vi "Config CCD.vi"(8 "error in (no error)":errorcluster, 11 "Configuration in":refnum<class "Configuration.lvclass">) -> (0 "error out":errorcluster, 3 "Configuration out":refnum<class "Configuration.lvclass">)   [LabVIEW 2016, in "CCD.lvlib" / "CCD Configuration.lvclass"]
uses:
  <userlib>/Common Components/Hardware/CCD/CCD Configuration.lvclass
  <userlib>/Configuration Dialog Actor/Configuration.lvclass
  <userlib>/Common Components/Hardware/CCD/CCD/camer data.ctl
  C:/Program Files (x86)/National Instruments/LabVIEW 2016/user.lib/Configuration Dialog Actor/Configuration.lvclass
  <userlib>/Common Components/Hardware/CCD/CCD Configuration.lvclass/CCD Configuration.ctl
  <userlib>/Common Components/Hardware/Abstract Hardware/Hardware.lvclass/Hardware.ctl
  <userlib>/Common Components/Hardware/CCD/CCD/CCD.lvclass/CCD.ctl
  <userlib>/Common Components/Hardware/DevInfo/DevInfo.lvclass/DevInfo.ctl
  <userlib>/Common Components/Hardware/Abstract Hardware/Read DevInfo.vi
  <userlib>/Common Components/Hardware/DevInfo/Read COMM Address.vi
  <userlib>/Common Components/Hardware/DevInfo/Read Sub-COMM Address.vi
  <userlib>/Common Components/Hardware/DevInfo/Read HW Type.vi
  <userlib>/Common Components/Hardware/DevInfo/Read Device Name.vi
  <userlib>/Common Components/Hardware/DevInfo/Read Status.vi
  <userlib>/Common Components/Hardware/CCD/CCD/CCD.lvclass
  C:/Program Files (x86)/National Instruments/LabVIEW 2016/user.lib/Common Components/Hardware/Abstract Hardware/Hardware.lvclass
  <userlib>/Common Components/Hardware/DevInfo/DevInfo.lvclass
panel:
  in  "Cluster":T1={"VideoMode"=0, "gain"=6818, "gamma"=0.43, "Contrast"=37.81818181818181, "Exposure"=32, "Saturation"=6818} {"Saturation" max=7764 scale=0.0..7764.0; "Exposure" scale=1.0..2048.0; "Contrast" min=0.0 max=78.0 scale=0.0..78.0 scale format="%.2f"; "gamma" min=0.43 max=5 scale=0.43..5.0; "gain" min=1000 max=7000 scale=1000.0..7000.0; "VideoMode" items=["640x480 RGB24 30FPS", "1024x768 RGB24 18FPS", "1920x1080 RGB24  10FPS", "2048x1536 RGB24 3FPS"]}
  out "Status":bool
  out "HW Type":string
  out "Sub-COMM Address":string
  out "COMM Address":string
  out "Device Name":string
  in  "Revert":bool
  in  "Apply":bool
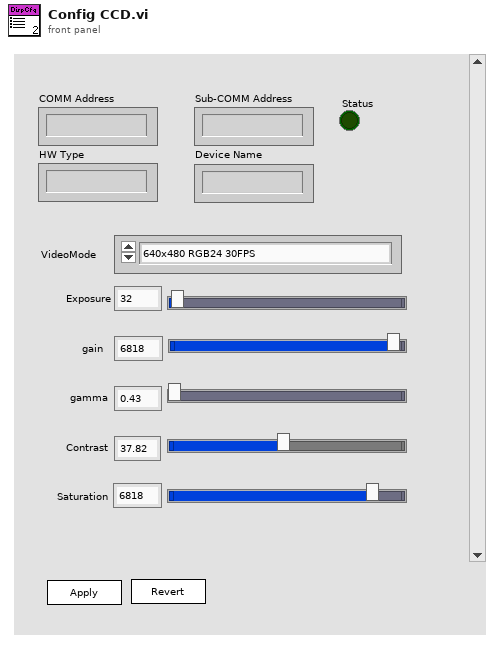
[diagram p1: front panel]
types:
  T1 = typedef "CCD.lvlib/CCD.lvclass/camer data.ctl" = cluster{"VideoMode":u16, "gain":u32, "gamma":sgl, "Contrast":dbl, "Exposure":u32, "Saturation":u32}
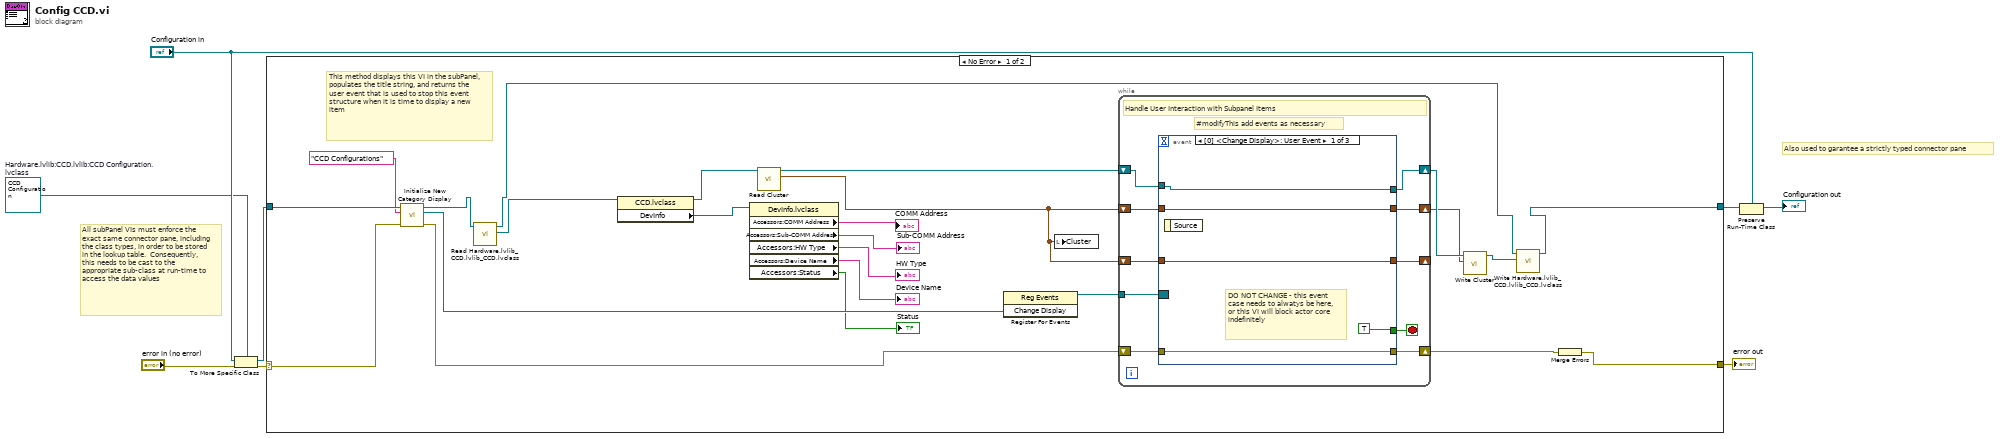
[diagram p0: block diagram]
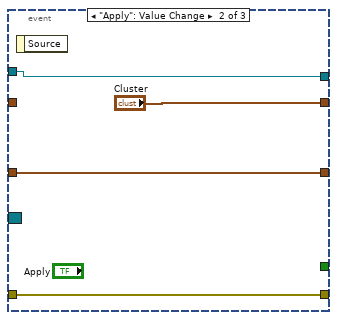
[diagram p2: hidden frame]
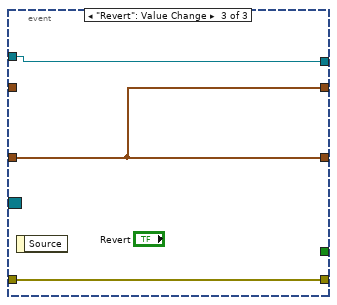
[diagram p3: hidden frame]
diagram:
  w1 = refnum<class "CCD Configuration.lvclass"> refnum  # Hardware.lvlib:CCD.lvlib:CCD Configuration.lvclass
  # "Also used to garantee a strictly typed connector pane"
  # "All subPanel VIs must enforce the exact same connector pane, including the class types, in order to be stored in the lookup table.  Consequently, this needs to be cast to the appropriate sub-class at run-time to access the data values"
  n1 = To More Specific Class(target class=w1, reference="Configuration in", error in="error in (no error)") -> (specific class reference=w6:refnum<class "CCD Configuration.lvclass">, error out=w2:errorcluster)
  n2 = case shown="No Error" w2 {
    selector: w2 -> [w28 w55]
    tunnel: w6 -> [w32 w56]
    tunnel: [w17 w56] -> w8
    tunnel: [w30 w55] -> w7
    frame No Error {
      # "This method displays this VI in the subPanel, populates the title string, and returns the user event that is used to stop this event structure when it is time to display a new item"
      n3 = call <userlib>:"Initialize New Category Display.vi"("error in (no error)"=w28, "Name to Display"="CCD Configurations", "Configuration in"=w32) -> ("error out"=w31:errorcluster, "Change Display"=w27:refnum<user-event>, "Configuration Out"=w18:refnum<class "CCD Configuration.lvclass">)  [unwired: 6 in]
      n4 = call <userlib>:"Read Hardware.lvlib_CCD.lvlib_CCD.lvclass.vi"("CCD Configuration in"=w18) -> ("Hardware.lvlib:CCD.lvlib:CCD.lvclass"=w15:refnum<class "CCD.lvclass">, "CCD Configuration out"=w16:refnum<class "CCD Configuration.lvclass">)  [unwired: 8 in, 1 out]
      n5 = property class="CCD.lvclass"(reference=w15) -> (reference out=w14:refnum<class "CCD.lvclass">, "DevInfo"=w21:refnum<class "DevInfo.lvclass">)  [unwired: 1 in, 1 out]
      n6 = property class="DevInfo.lvclass"(reference=w21) -> ("Accessors:COMM Address"=→"COMM Address":string, "Accessors:Sub-COMM Address"=→"Sub-COMM Address":string, "Accessors:HW Type"=→"HW Type":string, "Accessors:Device Name"=→"Device Name":string, "Accessors:Status"=→"Status":bool)  [unwired: 1 in, 2 out]
      n7 = call <userlib>:"Read Cluster.vi"("CCD in"=w14) -> ("Cluster"=w12:T1, "CCD out"=w13:refnum<class "CCD.lvclass">)  [unwired: 8 in, 1 out]
      n8 = register-events(w27) -> (reference out=w20:refnum<event-registration>)  [unwired: 2 in, 1 out]
      n9 = local write "Cluster"(w12) -> ()
      n10 = while {
        tunnel: w20 -> [w41]
        shift-right: [w40] -> w19
        shift-left: w31 -> [w39]
        shift-right: [w37] -> w11
        shift-left: w13 -> [w38]
        shift-right: [w35] -> w9
        shift-left: w12 -> [w36]
        shift-right: [w33] -> _
        shift-left: w12 -> [w34]
        stop <- w42 stop-if-true
        # "#modifyThis add events as necessary"
        # "Handle User Interaction with Subpanel Items"
        n11 = event shown="[0] <Change Display>: User Event" {
          selector: w41 -> [_ _ _]
          dyn-events: _ -> [_ _ _]
          timeout: _ -> [_ _ _]
          tunnel: [TRUE _ _] -> w42
          tunnel: [w46 w51 w54] -> w40
          tunnel: w39 -> [w46 w51 w54]
          tunnel: w38 -> [w45 w50 w52]
          tunnel: [w45 w50 w52] -> w37
          tunnel: w36 -> [w44 _ _]
          tunnel: [w44 "Cluster" w53] -> w35
          tunnel: w34 -> [w43 w48 w53]
          tunnel: [w43 w48 w53] -> w33
          event User Event {
            # "DO NOT CHANGE - this event case needs to alwatys be here, or this VI will block actor core indefinitely"
            n12 = event-data() -> ()  [unwired: 1 in, 1 out]
          }
          event "Apply": Value Change {
            n13 = event-data() -> ()  [unwired: 1 in, 1 out]
          }
          event "Revert": Value Change {
            n14 = event-data() -> ()  [unwired: 1 in, 1 out]
          }
        }
      }
      n15 = call <userlib>:"Write Cluster.vi"("Cluster"=w9, "CCD in"=w11) -> ("CCD out"=w10:refnum<class "CCD.lvclass">)  [unwired: 8 in, 1 out]
      n16 = call <userlib>:"Write Hardware.lvlib_CCD.lvlib_CCD.lvclass.vi"("Hardware.lvlib:CCD.lvlib:CCD.lvclass"=w10, "CCD Configuration in"=w16) -> ("CCD Configuration out"=w17:refnum<class "CCD Configuration.lvclass">)  [unwired: 8 in, 1 out]
      n17 = Merge Errors(w19) -> (w30:errorcluster)
    }
    frame Error {
    }
  }
  "error out" <- w7
  n18 = Preserve Run-Time Class(object in=w8, 2:"Configuration in") -> (object out=→"Configuration out":refnum<class "Configuration.lvclass">)  [unwired: 1 in, 1 out]
